vi "GE 5565PIORC.DMA.Block.In-Place Read (String).vi"(7 "bytes to read (-1: all)":i32=-1, 8 "error in (no error)":errorcluster, 9 "data in":string, 10 "Block Descriptor in":T1 {"descriptor params"."data ptr (lower)" format="%.0x"; "descriptor params"."data ptr (upper)" format="%.0x"; "descriptor params"."data size" format="%.0x"; "descriptor params"."next descriptor ptr" format="%.0x"; "descriptor size" format="%08x"; "descriptor ptr (RFM)" format="%08x"; "descriptor ptr (VISA)" format="%08x"}, 11 "GE 5565PIORC in":refnum<class "GE 5565PIORC.lvclass">) -> (0 "error out":errorcluster, 1 "data out":string, 2 "Block Descriptor out":T1 {"descriptor params"."data ptr (lower)" format="%.0x"; "descriptor params"."data ptr (upper)" format="%.0x"; "descriptor params"."data size" format="%.0x"; "descriptor params"."next descriptor ptr" format="%.0x"; "descriptor size" format="%08x"; "descriptor ptr (RFM)" format="%08x"; "descriptor ptr (VISA)" format="%08x"}, 3 "GE 5565PIORC out":refnum<class "GE 5565PIORC.lvclass">)   [LabVIEW 2016, in "GE 5565PIORC.lvclass"]
doc: "Reads <b>bytes to read</b> from the block specified by <B>Block Descriptor</B> and returns that bytes in <b>data</b>. The number of elements transferred will be either <B>bytes to read</B> or the number of bytes in <B>data</B>, whichever is smaller."
uses:
  GE 5565PIORC.lvclass
  Typedefs/GE 5565PIORC.Typedef.DMA Block Descriptor.ctl
  Typedefs/GE 5565PIORC.Typedef.DMA Block Descriptor Params.ctl
  <vilib>/Instr/_visa.llb/VISA Register Access Address Space.ctl
  GE 5565PIORC.lvclass/GE 5565PIORC.ctl
  GE 5565PIORC.VISA.Return Handler.vi
  <vilib>/Utility/error.llb/Error Cluster From Error Code.vi
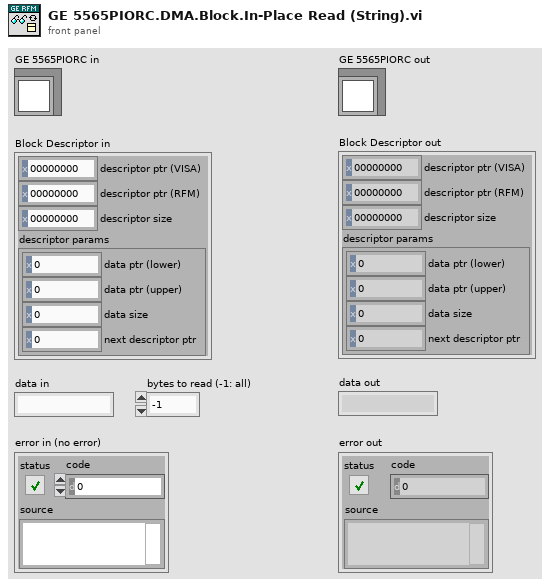
[diagram p1: front panel]
types:
  T1 = typedef "GE 5565PIORC.lvclass/GE 5565PIORC.Typedef.DMA Block Descriptor.ctl" = cluster{"descriptor ptr (VISA)":u32, "descriptor ptr (RFM)":u32, "descriptor size":u32, "descriptor params":T2}
  T2 = typedef "GE 5565PIORC.lvclass/GE 5565PIORC.Typedef.DMA Block Descriptor Params.ctl" = cluster{"data ptr (lower)":u32, "data ptr (upper)":u32, "data size":u32, "next descriptor ptr":u32}
  T3 = typedef "VISA Register Access Address Space.ctl" = u16
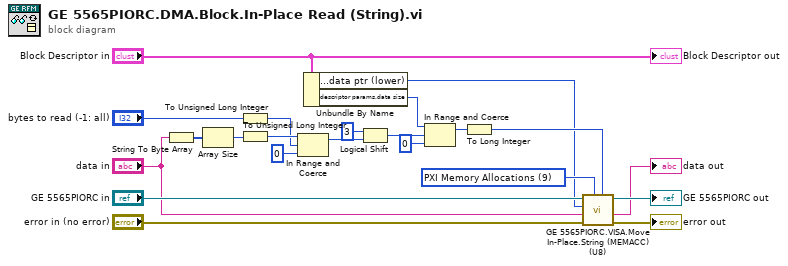
[diagram p0: block diagram]
diagram:
  w17 = T3 9 items=["VXI/VME A16"=1, "VXI/VME A24"=2, "VXI/VME A32"=3, "VXI/VME A64"=4, "PXI Memory Allocations"=9, "PXI Configuration"=10, "PXI BAR0"=11, "PXI BAR1"=12, "PXI BAR2"=13, "PXI BAR3"=14, "PXI BAR4"=15, "PXI BAR5"=16] ("address space")
  n1 = String To Byte Array(string="data in") -> (unsigned byte array=w4:u8[])
  n2 = Array Size(array=w4) -> (size(s)=w20:i32)
  n3 = To Unsigned Long Integer(number="bytes to read (-1: all)") -> (unsigned 32bit integer=w11:u32)
  n4 = To Unsigned Long Integer(number=w20) -> (unsigned 32bit integer=w16:u32)
  n5 = In Range and Coerce(upper limit=w16, x=w11, lower limit=u32 0) -> (coerced(x)=w15:u32)  [unwired: 1 out]
  n6 = Unbundle By Name("Block Descriptor in") -> ("descriptor params.data ptr (lower)"=w5:u32, "descriptor params.data size"=w12:u32)
  n7 = Logical Shift(y=i16 3, x=w15) -> (x << y=w14:u32)
  n8 = In Range and Coerce(upper limit=w12, x=w14, lower limit=u32 0) -> (coerced(x)=w9:u32)  [unwired: 1 out]
  n9 = To Long Integer(number=w9) -> (32bit integer=w8:i32)
  n10 = call "GE 5565PIORC.VISA.Move In-Place.String (MEMACC) (U8).vi"("count (-1: all)"=w8, "address space"=w17, "error in (no error)"="error in (no error)", "data in"="data in", "offset"=w5, "GE 5565PIORC in"="GE 5565PIORC in") -> ("error out"=→"error out":errorcluster, "data out"=→"data out":string, "GE 5565PIORC out"=→"GE 5565PIORC out":refnum<class "GE 5565PIORC.lvclass">)  [unwired: 3 in]
  "Block Descriptor out" <- "Block Descriptor in"
